vi "Sig2MS Init.vi"(8 "error in (no error)":errorcluster, 10 "signal in":waveform(sgl), 11 "Sig2MS in":refnum<class "Sig2MS.lvclass">) -> (0 "error out":errorcluster, 2 "Size":i32, 3 "Sig2MS out":refnum<class "Sig2MS.lvclass">)   [LabVIEW 2018, in "Sig2MS.lvclass"]
uses:
  Sig2MS.lvclass
  Sig2MS.lvclass/Sig2MS.ctl
  Overload/Experiment Condition/_PC_Pub_ExpCondiValue_SignalRemarks.vi
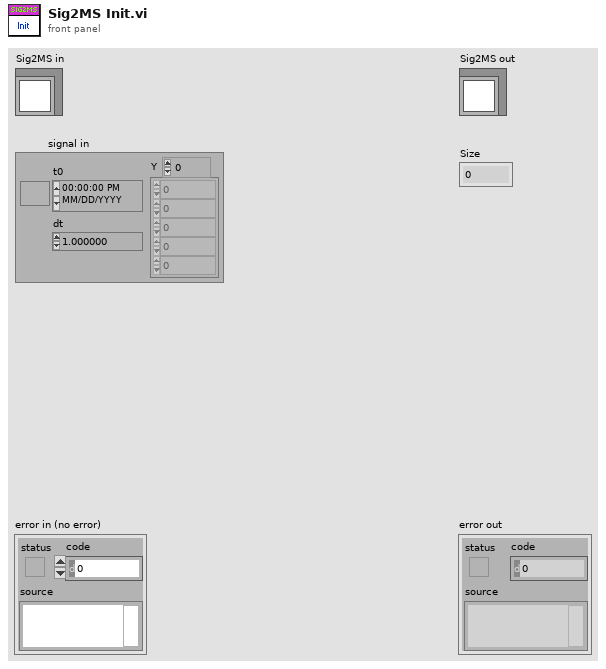
[diagram p1: front panel]
types:
  T1 = cluster{"priDt":dbl, "priXData":dbl[], "priYData":sgl[], "beta":dbl[]}[]
  T2 = cluster{"InfoID":u64, "SignalInfo":cluster{"Label":string, "dt":dbl, "Length":u32, "RefVolt":dbl, "mzTable":cluster{"t":dbl[], "mz":dbl[], "beta":dbl[]}}[]}
  T3 = cluster{"Label":string, "dt":dbl, "Length":u32, "RefVolt":dbl, "mzTable":cluster{"t":dbl[], "mz":dbl[], "beta":dbl[]}}[]
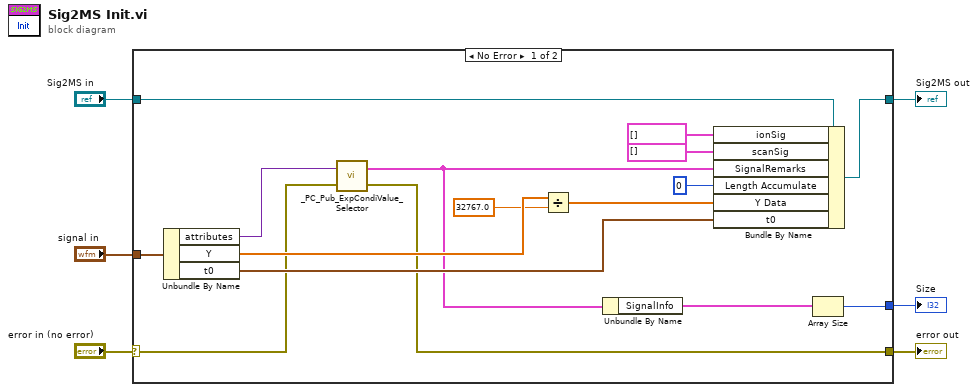
[diagram p0: block diagram]
diagram:
  n1 = case shown="No Error" "error in (no error)" {
    selector: "error in (no error)" -> [w10 w24]
    tunnel: [w11 w24] -> w5
    tunnel: [w19 w23] -> w3
    tunnel: "Sig2MS in" -> [w20 w23]
    tunnel: "signal in" -> [w22 _]
    tunnel: [w14 _] -> w1
    frame No Error {
      n2 = Unbundle By Name(w22) -> ("attributes"=w9:variant, "Y"=w21:sgl[], "t0"=w15:timestamp)
      n3 = call-poly "_PC_Pub_ExpCondiValue_Selector.vi"("error in (no error)"=w10, "expCondiVariant"=w9) -> ("error out"=w11:errorcluster, "SignalRemarks"=w13:T2)
      n4 = Divide(x=w21, y=sgl 32767.0) -> (x/y=w16:sgl[])
      n5 = Unbundle By Name(w13) -> ("SignalInfo"=w12:T3)
      n6 = Bundle By Name(cluster=w20, "ionSig"=cluster{"secDt":dbl, "secYData":sgl[]}[] [], "scanSig"=T1 [], "SignalRemarks"=w13, "Length Accumulate"=u32 0, "Y Data"=w16, "t0"=w15) -> (w19:refnum<class "Sig2MS.lvclass">)
      n7 = Array Size(array=w12) -> (size(s)=w14:i32)
    }
    frame Error {
    }
  }
  "error out" <- w5
  "Sig2MS out" <- w3
  "Size" <- w1
